vi "BarLIV_Ex_DataOut_autoReport.vi"(2 "error in (no error)":errorcluster, 3 "Bar_LIV_AutoRep":path=path "D:/LabVIEW_prog/Trumpf_Database_Connect/DM17_TestFiles_AutoReport/30082943autoreport_Pre_05-31-2019_10-11-46.xlsx") -> (0 "error out":errorcluster={"status"=TRUE, "code"=7, "source"="NI_Excel.lvclass:new report subVI.vi -> NI_report.lvclass:New Report.vi -> BarLIV_Ex_DataOut_autoReport.vi\r\n"}, 1 "BarLIV AutoRep Output":T1={"Date"="12/30/1899", "LIV Data"=[], "Polarization"=0.0, "Bar SN"="", "Bar WO"="", "Wafer ID"=""})   [LabVIEW 2017]
uses:
  <vilib>/addons/_office/excel.llb/Excel Get Data (str).vi
  <vilib>/addons/_office/excel.llb/Excel Get Data ([dbl]).vi
  <vilib>/addons/_office/excel.llb/Excel Get Data (dbl).vi
  <vilib>/Utility/NIReport.llb/NI_report.lvclass
  <vilib>/addons/_office/NI_ReportGenerationToolkit.lvlib
  <vilib>/Utility/NIReport.llb/Excel/NI_Excel.lvclass
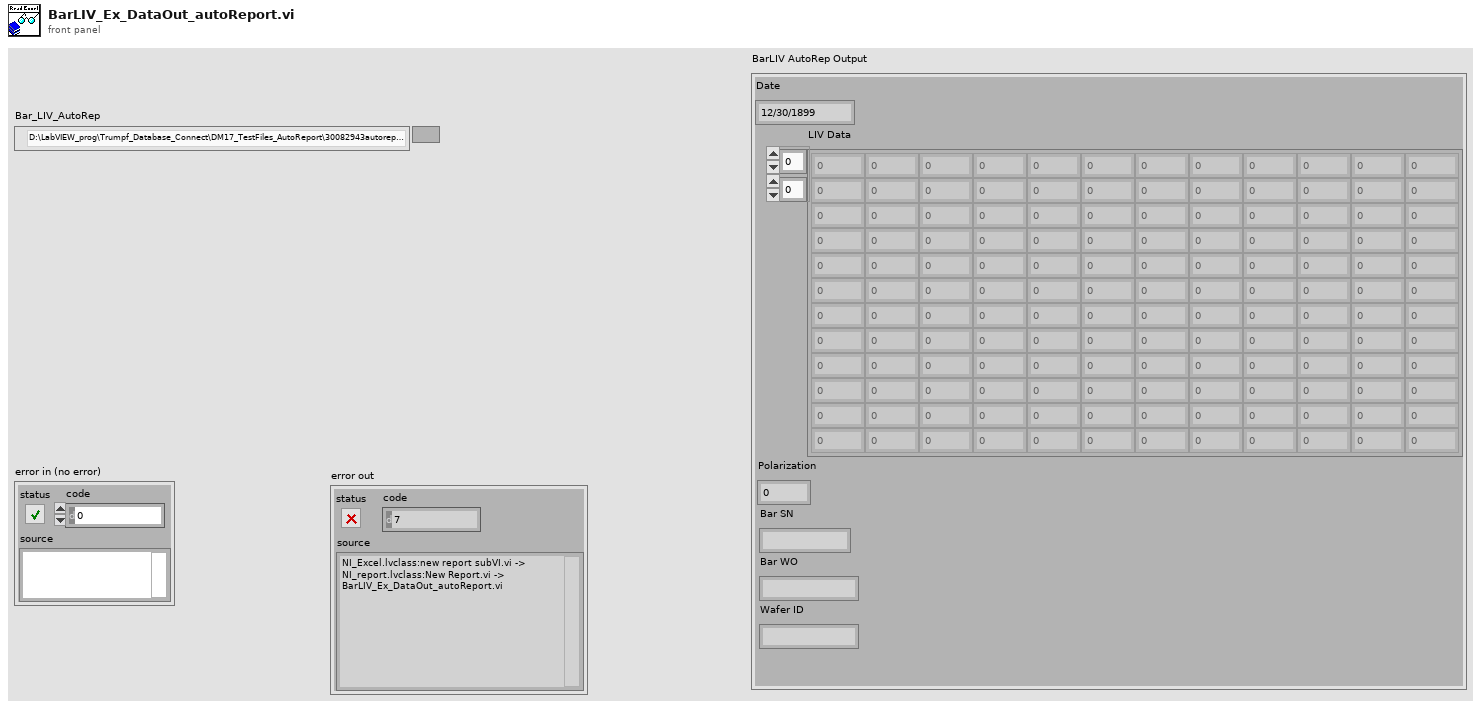
[diagram p1: front panel]
types:
  T1 = cluster{"Date":string, "LIV Data":dbl[][], "Polarization":dbl, "Bar SN":string, "Bar WO":string, "Wafer ID":string}
  T2 = enum16{"Standard Report", "HTML", "Word", "Excel"}
  T3 = cluster{"date/time string":string, "data":dbl[][], dbl, "data":string, "data":string, "data":string}
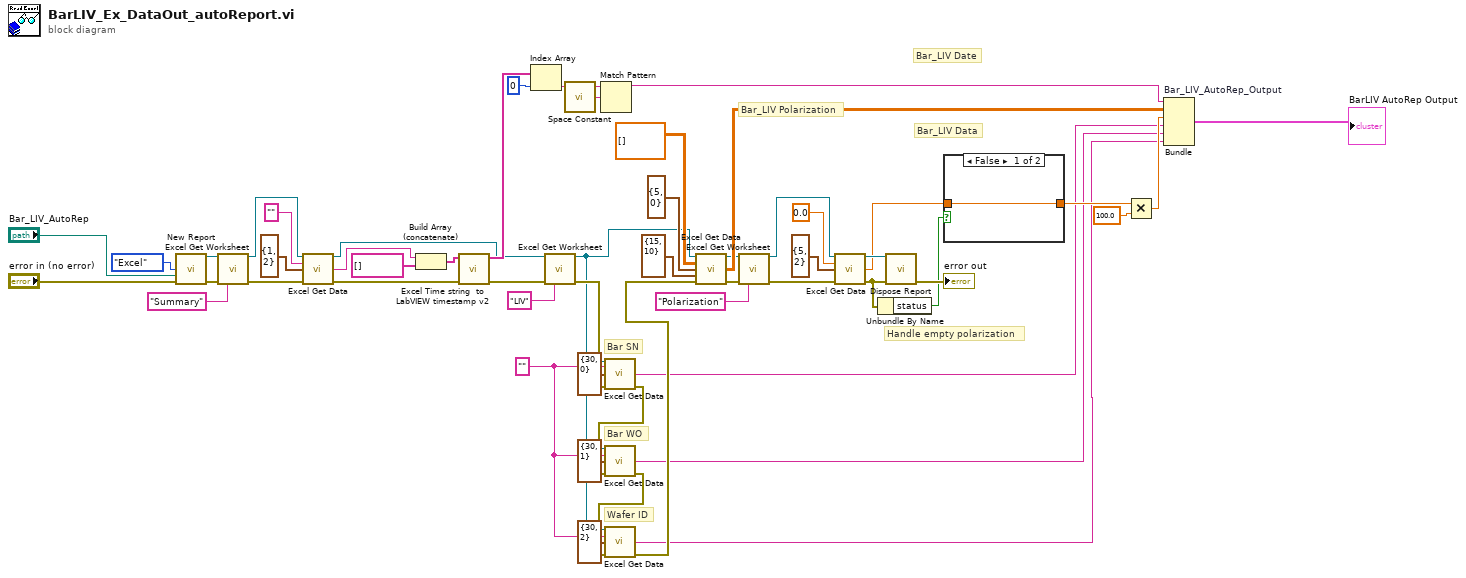
[diagram p0: block diagram]
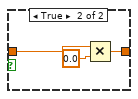
[diagram p2: hidden frame]
diagram:
  w13 = ""
  # "Wafer ID"
  # "Bar WO"
  # "Bar SN"
  # "Handle empty polarization"
  # "Bar_LIV Polarization"
  # "Bar_LIV Date"
  # "Bar_LIV Data"
  n1 = call <vilib>:"New Report.vi"("report type"=T2."Excel", "template (empty)"="Bar_LIV_AutoRep", "error in (no error)"="error in (no error)") -> ("report out"=w52:refnum<class "NI_report.lvclass">, "error out"=w51:errorcluster)  [unwired: 11 in]
  n2 = call <vilib>:"Excel Get Worksheet.vi"("report in"=w52, "error in (no error)"=w51, "name (\"\")"="Summary" ("name (\"\")")) -> ("report out"=w49:refnum<class "NI_report.lvclass">, "error out"=w47:errorcluster)  [unwired: 1 in, 10 out]
  n3 = call-poly <vilib>:"Excel Get Data.vi"("report in"=w49, "data type"="", "start (0, 0)"=cluster{"start row":i32, "start column":i32} {"start row"=1, "start column"=2}, "error in (no error)"=w47) -> ("report out"=w39:refnum<class "NI_report.lvclass">, "data"=w44:string, "error out"=w42:errorcluster)  [unwired: 9 in]
  n4 = Build Array (concatenate)(w44, string[] []) -> (w43:string[])
  n5 = call "Excel Time string  to LabVIEW timestamp v2.vi"("Error In"=w42, "XLDateIn"=w43) -> ("Error Out"=w38:errorcluster, "DateOut"=w40:string[])  [unwired: 7 in, 1 out]
  n6 = Index Array(array=w40, index=0) -> (element=w20:string)
  n7 = call <vilib>:"Excel Get Worksheet.vi"("report in"=w39, "error in (no error)"=w38, "name (\"\")"="LIV" ("name (\"\")")) -> ("report out"=w2:refnum<class "NI_report.lvclass">, "error out"=w9:errorcluster)  [unwired: 1 in, 10 out]
  n8 = call <vilib>:"Space Constant.vi"() -> ("String"=w19:string)
  n9 = Match Pattern(string=w20, regular expression=w19) -> (before substring=w18:string)  [unwired: 1 in, 3 out]
  n10 = call-poly <vilib>:"Excel Get Data.vi"("report in"=w2, "data type"=w13, "start (0, 0)"=cluster{"start row":i32, "start column":i32} {"start row"=30, "start column"=0}, "error in (no error)"=w9) -> ("data"=w5:string, "error out"=w8:errorcluster)  [unwired: 9 in, 1 out]
  n11 = call-poly <vilib>:"Excel Get Data.vi"("report in"=w2, "data type"=w13, "start (0, 0)"=cluster{"start row":i32, "start column":i32} {"start row"=30, "start column"=1}, "error in (no error)"=w8) -> ("data"=w4:string, "error out"=w7:errorcluster)  [unwired: 9 in, 1 out]
  n12 = call-poly <vilib>:"Excel Get Data.vi"("report in"=w2, "data type"=w13, "start (0, 0)"=cluster{"start row":i32, "start column":i32} {"start row"=30, "start column"=2}, "error in (no error)"=w7) -> ("data"=w3:string, "error out"=w6:errorcluster)  [unwired: 9 in, 1 out]
  n13 = call-poly <vilib>:"Excel Get Data.vi"("report in"=w2, "data type"=dbl[][] [], "start (-1, -1)"=cluster{"row":i32, "column":i32} {"row"=5, "column"=0}, "end (-1, -1)"=cluster{"row":i32, "column":i32} {"row"=15, "column"=10}, "error in (no error)"=w6) -> ("report out"=w32:refnum<class "NI_report.lvclass">, "data"=w33:dbl[][], "error out"=w31:errorcluster)  [unwired: 8 in]
  n14 = call <vilib>:"Excel Get Worksheet.vi"("report in"=w32, "error in (no error)"=w31, "name (\"\")"="Polarization" ("name (\"\")")) -> ("report out"=w29:refnum<class "NI_report.lvclass">, "error out"=w26:errorcluster)  [unwired: 1 in, 10 out]
  n15 = call-poly <vilib>:"Excel Get Data.vi"("report in"=w29, "data type"=0.0, "start (0, 0)"=cluster{"row":i32, "column":i32} {"row"=5, "column"=2} ("start (-1, -1)"), "error in (no error)"=w26) -> ("report out"=w25:refnum<class "NI_report.lvclass">, "data"=w15:dbl, "error out"=w17:errorcluster)  [unwired: 9 in]
  n16 = Unbundle By Name(w17) -> ("status"=w16:bool)
  n17 = call-dynamic "Dispose Report.vi"("report in"=w25, "error in (no error)"=w17) -> ("error out"=→"error out":errorcluster)  [unwired: 13 in]
  n18 = case shown="False" w16 {
    tunnel: w15 -> [w55 w58]
    tunnel: [w55 w56] -> w14
    frame False {
    }
    frame True {
      n19 = Multiply(x=w58, y=0.0) -> (x*y=w56:dbl)
    }
  }
  n20 = Multiply(x=w14, y=100.0) -> (x*y=w22:dbl)
  n21 = Bundle "Bar_LIV_AutoRep_Output"("date/time string"=w18, "data"=w33, w22, "data"=w5, "data"=w4, "data"=w3) -> (→"BarLIV AutoRep Output":T3)  [unwired: 1 in]
